vi "Node - Handshaking Test.vi"() -> ()   [LabVIEW 2016]
uses:
  <vilib>/pximc/Initialize Writer Session (U32).vi
  <vilib>/pximc/Connect (U32).vi
  <vilib>/pximc/Write (U32).vi
  PXImc Router.lvlib
  <vilib>/pximc/nipximc.lvlib
panel:
  out "error out 2":errorcluster caption="error out"
  in  "Connection Timeout (s)":dbl
  in  "Data In 2":u32[](array[numeric])
  in  "Resource Name In":string
  in  "Writer Conn ID":u16
  out "error out":errorcluster
  in  "Data In":u32[](array[numeric])
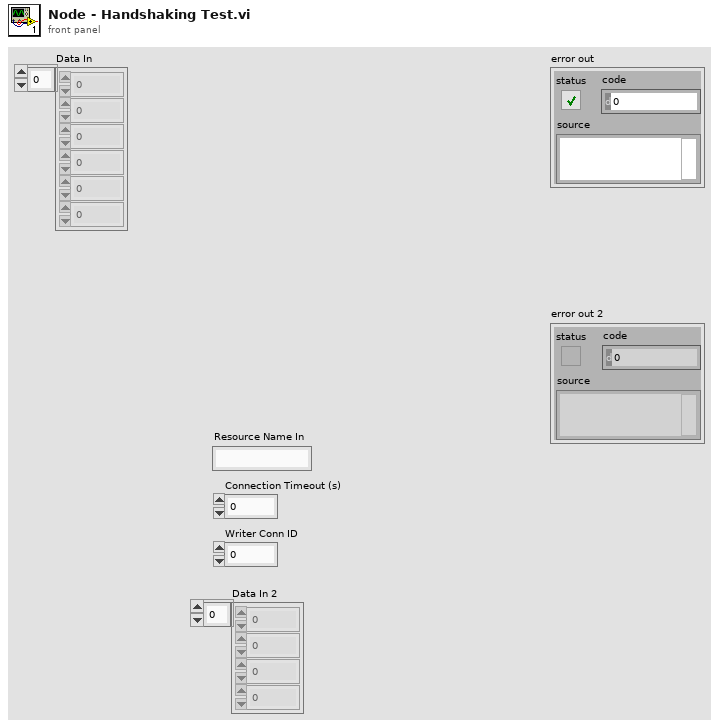
[diagram p1: front panel]
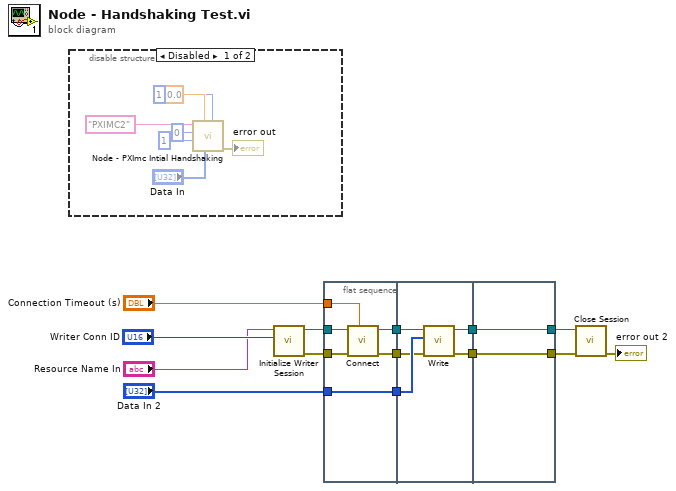
[diagram p0: block diagram]
diagram:
  n1 = disable-structure shown="Disabled" {
    frame Disabled {
      n2 = call "Node - PXImc Intial Handshaking.vi"("Reader Buffer Size In"=u64 1, "Data In"="Data In", "Connection Timeout (s)"=60.0, "Reader Conn ID"=u16 1, "Writer Conn ID"=u16 0, "Resource Name In"="PXIMC2") -> ("error out"=→"error out":errorcluster)  [unwired: 5 in]
    }
    frame Enabled {
    }
  }
  n3 = call-poly <vilib>:"Initialize Writer Session.vi"("connection id (1)"="Writer Conn ID", "interface"="Resource Name In") -> ("error out"=w4:errorcluster, "session out"=w3:refnum<k21>)  [unwired: 8 in]
  n4 = flat-sequence {
    tunnel: w3 -> [w27]
    tunnel: w4 -> [w26]
    tunnel: [w25] -> w14
    tunnel: [w24] -> w13
    tunnel: "Connection Timeout (s)" -> [w22]
    tunnel: "Data In 2" -> [w23]
    tunnel: [w23] -> w12
    tunnel: w14 -> [w32]
    tunnel: w13 -> [w28]
    tunnel: [w31] -> w11
    tunnel: [w30] -> w10
    tunnel: w12 -> [w29]
    tunnel: [w33] -> w6
    tunnel: [w34] -> w5
    tunnel: w11 -> [w34]
    tunnel: w10 -> [w33]
    frame #0 {
      n5 = call-poly <vilib>:"Connect.vi"("timeout in seconds (-1)"=w22, "error in (no error)"=w26, "session in"=w27) -> ("error out"=w24:errorcluster, "session out"=w25:refnum<k21>)  [unwired: 7 in]
    }
    frame #1 {
      n6 = call-poly <vilib>:"Write.vi"("error in (no error)"=w28, "data"=w29, "session in"=w32) -> ("error out"=w30:errorcluster, "session out"=w31:refnum<k21>)  [unwired: 6 in, 1 out]
    }
    frame #2 {
    }
  }
  n7 = call <vilib>:"Close Session.vi"("error in (no error)"=w6, "session in"=w5) -> ("error out"=→"error out 2":errorcluster)  [unwired: 9 in]
